vi "FROG_FFT.vi"(3 "Time Delay Resolution":u16, 5 "Signal":T2) -> (1 "Fit Trace":dbl[][](array[numeric]), 2 "Complex Electric Field":cdb[][](array[numeric]))   [LabVIEW 2013]
uses:
  <vilib>/Analysis/2dsp.llb/Complex FFT.vi
  <vilib>/Analysis/baseanly.llb/Quick Scale 2D.vi
  <vilib>/Analysis/2dsp.llb/1D Cross Correlation (DBL).vi
  <vilib>/Analysis/NI_AALPro.lvlib
  <vilib>/Analysis/NI_AALBase.lvlib
  <vilib>/gmath/NI_Gmath.lvlib
panel:
  in  "milliseconds to wait":u32=1
  out "Result":cluster{"Time Array":ext[], dbl[]}(graph)
  in  "Debug":bool
  out "Debug":T1(graph)
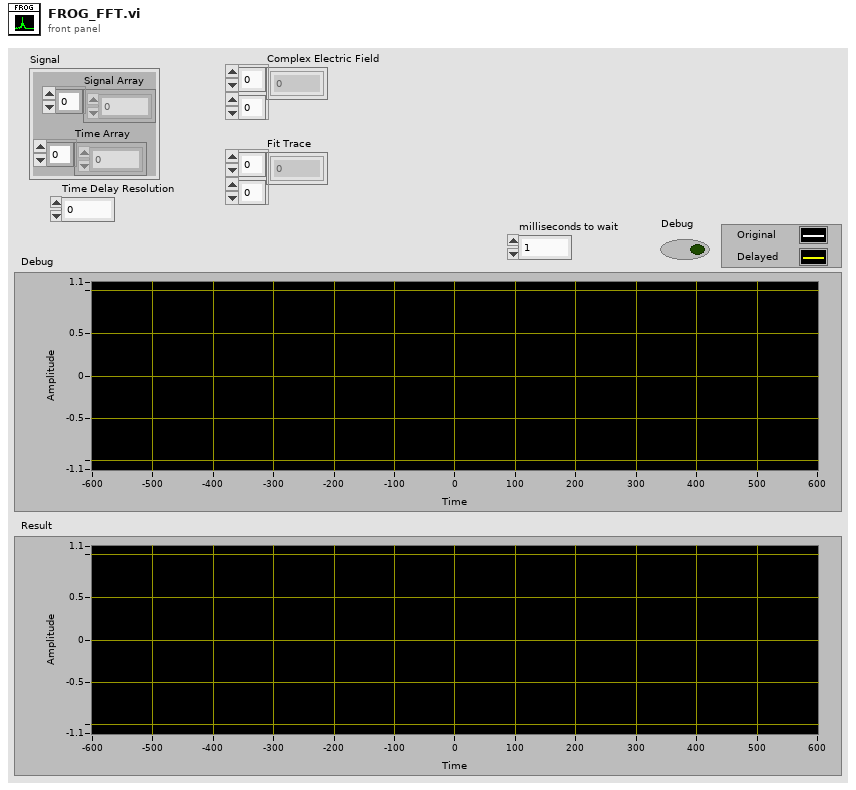
[diagram p1: front panel]
types:
  T1 = cluster{"Time Array":ext[], "Signal Array":dbl[]}[]
  T2 = cluster{"Signal Array":dbl[], "Time Array":ext[]}
  T3 = cluster{"Time Array":ext[], "Signal Array":dbl[]}
  T4 = cluster{"Time Array":ext[], "Signal Array":cdb[]}[]
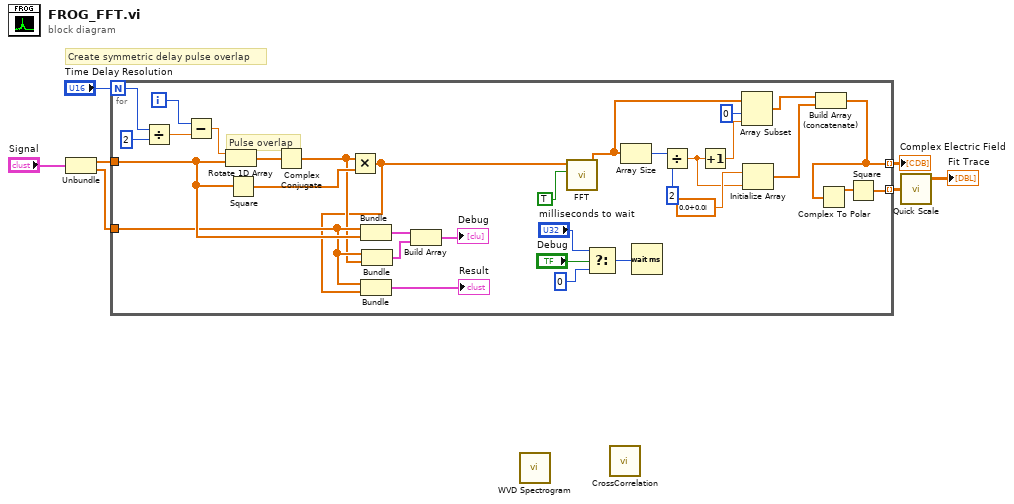
[diagram p0: block diagram]
diagram:
  # "Create symmetric delay pulse overlap"
  n1 = Unbundle("Signal") -> ("Signal Array"=w6:dbl[], "Time Array"=w1:ext[])
  n2 = for {
    N: "Time Delay Resolution" -> [w39]
    tunnel: w6 -> [w30]
    tunnel: [w8] -> w7 mode=indexing
    tunnel: [w36] -> w3 mode=indexing
    tunnel: w1 -> [w22]
    i -> [w33]
    # "Pulse overlap"
    n3 = Divide(x=w39, y=2) -> (x/y=w34:dbl)
    n4 = Subtract(x=w33, y=w34) -> (x-y=w32:dbl)
    n5 = Rotate 1D Array(1:w30, 2:w32) -> (0:w20:dbl[])
    n6 = Square(x=w30) -> (x^2=w31:dbl[])
    n7 = Complex Conjugate(1:w20) -> (0:w19:cdb[])
    n8 = Multiply(x=w19, y=w31) -> (x*y=w18:cdb[])
    n9 = Bundle("Time Array"=w22, "Signal Array"=w30) -> (w29:T3)  [unwired: 1 in]
    n10 = Bundle("Time Array"=w22, w18) -> (→"Result":cluster{"Time Array":ext[], cdb[]})  [unwired: 1 in]
    n11 = Bundle("Time Array"=w22, w19) -> (w28:cluster{"Time Array":ext[], cdb[]})  [unwired: 1 in]
    n12 = Build Array(w29, w28) -> (→"Debug":T4)
    n13 = call-poly <vilib>:"FFT.vi"("shift?"=TRUE, "X"=w18) -> ("FFT {X}"=w9:cdb[])  [unwired: 8 in, 1 out]
    n14 = Select(t="milliseconds to wait", s="Debug", f=u32 0) -> (s? t:f=w25:u32)
    n15 = Array Size(array=w9) -> (size(s)=w17:i32)
    n16 = Wait (ms)(milliseconds to wait=w25) -> ()  [unwired: 1 out]
    n17 = Divide(x=w17, y=2) -> (x/y=w11:dbl)
    n18 = Increment(x=w11) -> (x+1=w10:dbl)
    n19 = Array Subset(array=w9, index=0, length=w10) -> (w15:cdb[])
    n20 = Initialize Array(cdb 0.0+0.0i, w11) -> (w14:cdb[])
    n21 = Build Array (concatenate)(w15, w14) -> (w8:cdb[])
    n22 = Complex To Polar(r * e^(i*theta)=w8) -> (r=w37:dbl[])  [unwired: 1 out]
    n23 = Square(x=w37) -> (x^2=w36:dbl[])
  }
  "Complex Electric Field" <- w7
  n24 = call <vilib>:"WVD Spectrogram.vi"() -> ()  [unwired: 2 in, 2 out]
  n25 = call-poly <vilib>:"CrossCorrelation.vi"() -> ()  [unwired: 10 in, 2 out]
  n26 = call-poly <vilib>:"Quick Scale.vi"("X"=w3) -> ("Yij=Xij/Max|X|"=→"Fit Trace":dbl[][])  [unwired: 2 out]
